vi "EvaluateCodeLine.vi"(10 "Timings":i32[](array[numeric]), 11 "input string":string) -> (2 "read":bool, 3 "timeout (ms)":i32)   [LabVIEW 2013]
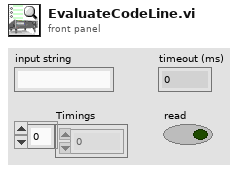
[diagram p1: front panel]
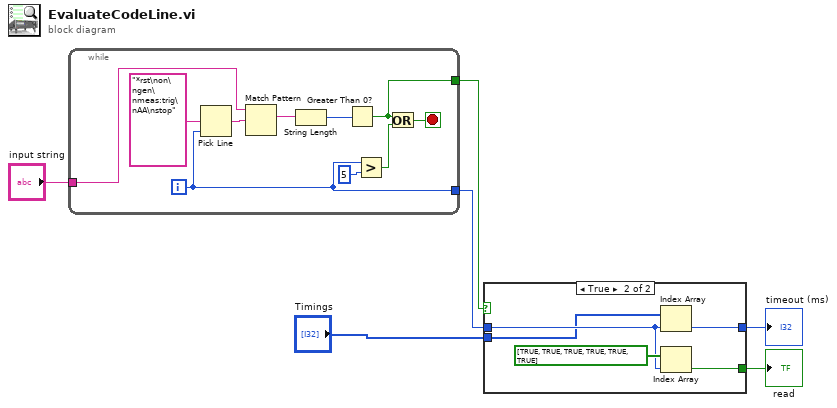
[diagram p0: block diagram]
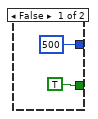
[diagram p2: hidden frame]
diagram:
  n1 = while {
    tunnel: "input string" -> [w8]
    tunnel: [w13] -> w1
    tunnel: [w9] -> w2
    i -> [w9]
    stop <- w12 stop-if-true
    n2 = Pick Line(multi-line string="*rst\non\ngen\nmeas:trig\nAA\nstop", line index=w9) -> (output string=w7:string)  [unwired: 1 in]
    n3 = Match Pattern(string=w8, regular expression=w7) -> (match substring=w16:string)  [unwired: 1 in, 3 out]
    n4 = String Length(string=w16) -> (length=w14:i32)
    n5 = Greater Than 0?(x=w14) -> (x > 0?=w13:bool)
    n6 = Greater?(x=w9, y=5) -> (0:w10:bool)
    n7 = Or(x=w13, y=w10) -> (x .or. y?=w12:bool)
  }
  n8 = case shown="True" w1 {
    tunnel: [500 ("timeout (ms)") w23] -> w3
    tunnel: w2 -> [_ w21]
    tunnel: [TRUE w20] -> w4
    tunnel: "Timings" -> [_ w19]
    frame False {
    }
    frame True {
      n9 = Index Array(array=w19, index=w21) -> (element=w23:i32)
      n10 = Index Array(array=bool[] [TRUE, TRUE, TRUE, TRUE, TRUE, TRUE], index=w21) -> (element=w20:bool)
    }
  }
  "read" <- w4
  "timeout (ms)" <- w3
